vi "7HP v2.0 external control - EnFlo_Specific.vi"(6 "Datalog file path (full)":path, 7 "COM port":refnum<visa-resource-name>, 8 "Log data stream":bool, 9 "Set data rate (Hz)":u8(ring)=14 items=["1", "2", "4", "5", "8", "10", "16", "20", "25", "32", "40", "50", "64", "80", "100", "125", "160", "200", "250", "320", "400", "500", "625", "800", "1000"], 10 "N samples":u32=1000, 11 "Command":T2="D") -> (0 "Error":errorcluster, 1 "Returned data rate (Hz)":u16, 2 "Serial number":sgl, 3 "Data out":T3[](array[typedef]) {"Time stamp" format="%<%.6X\n%x>T"}, 4 "Rendezvous out":bool)   [LabVIEW 2021]
doc: "7HP test and configuration software.\nVersion 2.0\nSurrey Sensors Ltd.\n11/2023"
uses:
  ctls/7HP_Cmd (USB).ctl
  ctls/7HP_Data cluster.ctl
  Globals/Meas_global.vi
panel:
  in  "COM port 2":refnum<visa-resource-name>
  in  "Main":T1(tab)
  out "Subsystems ok":bool[](array[boolean])
  out "Pressure sensor values in range":bool[](array[boolean])
  out "Pressure sensor temperatures in range":bool[](array[boolean])
  out "Pressure sensor EEPROM checksums ok":bool[](array[boolean])
  out "P_raw_Azero":sgl[](array[numeric])
  out "n":u16
  out "Auto zero progBar":u16(slide) caption="Collecting samples, please maintain dP = 0" scale=0.0..1000.0
  out "Neural network binary (read-only)":string
  out "ANN checksum ok":bool
  out "Neural network checksum":u16 format="%04x"
  in  "EEPROM array 2":u16[](array[numeric])
  in  "EEPROM array":sgl[](array[numeric]) format="%#.3f"
  out "EEPROM checksum ok":bool
  out "EEPROM checksum":u16 format="%04x"
  out "received":bool
  out "sent":bool
  out "Neural network outputs":sgl[](array[numeric]) format="%#.2f"
  out "Frame errors":u32
  out "Checksum errors":u32
  in  "Stop Data":bool
  out "Rel. humidity (%)":sgl format="%#.2f"
  out "T_board (°C)":sgl format="%#.2f"
  out "T_external (°C)":sgl format="%#.2f"
  out "P_atmos (mbar)":sgl format="%#.2f"
  out "Checksum ok":bool
  out "Gyration vector (° / s)":sgl[](array[numeric]) format="%#.3f"
  out "Acceleration vector (g)":sgl[](array[numeric]) format="%#.3f"
  out "Pressures":sgl[][](graph)
  out "Stream enabled":bool
  out "Pitch (°)":sgl format="%.2f"
  out "Roll (°)":sgl format="%.2f"
  # "Paul Nathan 11/2023"
  # "Pressure sensor 0 EEPROM checksum okay"
  # "Pressure sensor 0 value in range"
  # "Pressure sensor 1 EEPROM checksum okay"
  # "Pressure sensor 1 value in range"
  # "Pressure sensor 2 EEPROM checksum okay"
  # "Pressure sensor 2 value in range"
  # "Pressure sensor 3 EEPROM checksum okay"
  # "Pressure sensor 3 value in range"
  # "Pressure sensor 4 EEPROM checksum okay"
  # "Pressure sensor 4 value in range"
  # "Pressure sensor 5 EEPROM checksum okay"
  # "Pressure sensor 5 value in range"
  # "Pressure sensor 6 EEPROM checksum okay"
  # "Pressure sensor 6 value in range"
  # "Environmental sensor present"
  # "Pressure sensor 0 temperature in range"
  # "Inertial sensor present"
  # "Pressure sensor 1 temperature in range"
  # "Accelerometer self test pass"
  # "Pressure sensor 2 temperature in range"
  # "Gyroscope self test pass"
  # "Pressure sensor 3 temperature in range"
  # "External thermistor value in range"
  # "Pressure sensor 4 temperature in range"
  # "MCU EEPROM checksum ok"
  # "Pressure sensor 5 temperature in range"
  # "Neural network enabled"
  # "Pressure sensor 6 temperature in range"
  # "Neural network integrity pass"
  # "%"
  # "P0 raw auto-zero"
  # "P1 raw auto-zero"
  # "P2 raw auto-zero"
  # "P3 raw auto-zero"
  # "P4 raw auto-zero"
  # "P5 raw auto-zero"
  # "P6 raw auto-zero"
  # "Power-up defaults"
  # "P0 raw auto-zero"
  # "Data rate (Hz)"
  # "P1 raw auto-zero"
  # "TTL streaming"
  # "P2 raw auto-zero"
  # "USB streaming"
  # "P3 raw auto-zero"
  # "TTL stream contains full data"
  # "P4 raw auto-zero"
  # "Accelerometer range mode"
  # "P5 raw auto-zero"
  # "Gyroscope range mode"
  # "P6 raw auto-zero"
  # "IMU rate mode"
  # "Atmospheric pressure offset (Pa)"
  # "HW trigger edge polarity"
  # "External thermistor temperature offset (°C)"
  # "Neural network enabled"
  # "Serial number"
  # "UVW coordinate system"
  # "TTL baud rate (bps)"
  # "Accelerometer vector magnitude scale factor"
  # "Gyroscope x component offset (deg / s)"
  # "Gyroscope y component offset (deg / s)"
  # "Gyroscope z component offset (deg / s)"
  # "||U|| (m/s)"
  # "Pitch (deg)"
  # "Yaw (deg)"
  # "U (m/s)"
  # "V (m/s)"
  # "W (m/s)"
  # "w_x"
  # "w_y"
  # "w_z"
  # "a_x"
  # "a_y"
  # "a_z"
  # "||U|| (m/s)"
  # "Pitch (deg)"
  # "Yaw (deg)"
  # "U (m/s)"
  # "V (m/s)"
  # "W (m/s)"
  # "w_x"
  # "w_y"
  # "w_z"
  # "a_x"
  # "a_y"
  # "a_z"
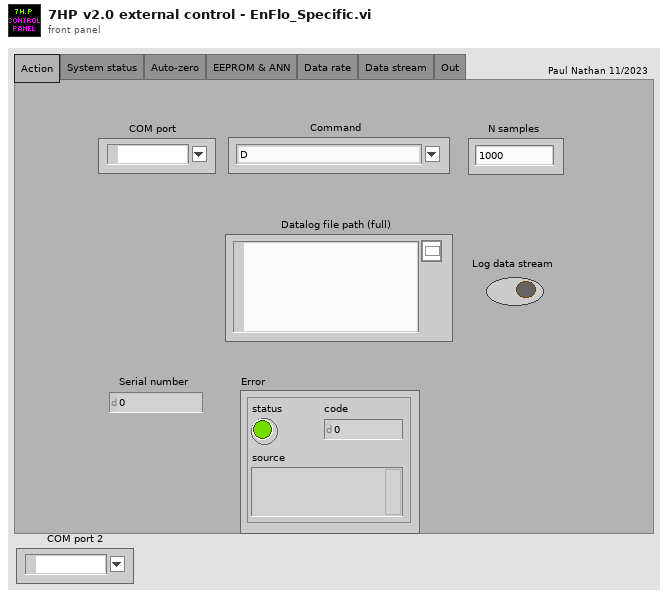
[diagram p1: front panel]
types:
  T1 = enum32{"Action", "System status", "Auto-zero", "EEPROM & ANN", "Data rate", "Data stream", "Out"}
  T2 = typedef "7HP_Cmd (USB).ctl" = string
  T3 = typedef "7HP_Data cluster.ctl" = cluster{"Time stamp":timestamp, "Pressures (Pa)":sgl[], "T_external (°C)":sgl, "P_atmos (mbar)":sgl, "T_board (°C)":sgl, "Rel. humidity (%)":sgl, "Acceleration vector (g)":sgl[], "Gyration vector (deg / s)":sgl[], "Neural network outputs":sgl[]}
  T4 = enum16{"open", "replace", "create", "open or create", "replace or create", "replace or create with confirmation"}
  T5 = typedef "Rendezvous RefNum" = refnum<k1>
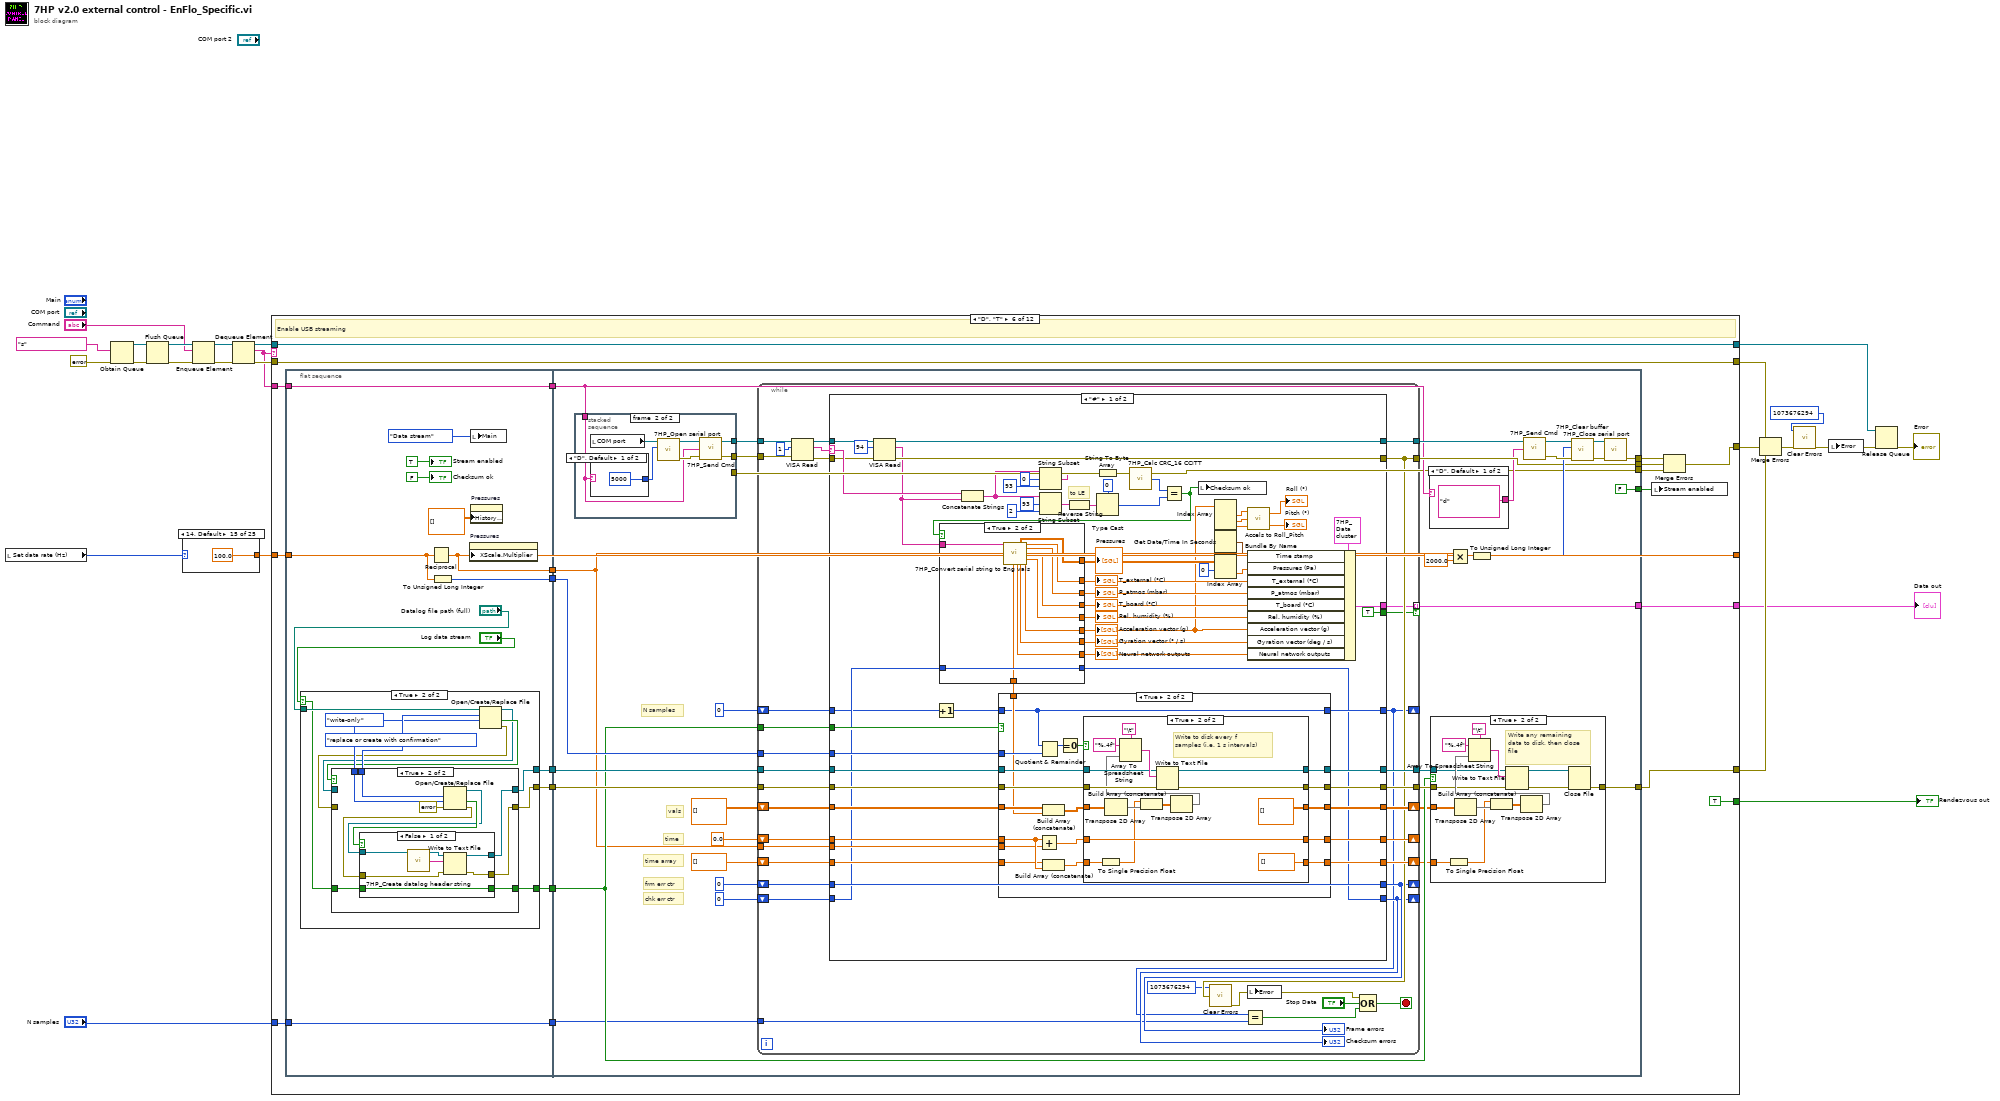
[diagram p0: block diagram]
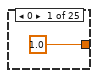
[diagram p2: hidden frame]
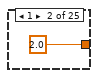
[diagram p3: hidden frame]
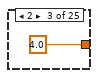
[diagram p4: hidden frame]
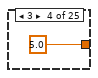
[diagram p5: hidden frame]
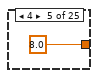
[diagram p6: hidden frame]
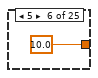
[diagram p7: hidden frame]
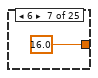
[diagram p8: hidden frame]
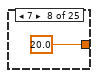
[diagram p9: hidden frame]
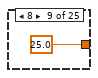
[diagram p10: hidden frame]
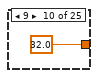
[diagram p11: hidden frame]
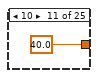
[diagram p12: hidden frame]
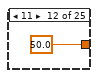
[diagram p13: hidden frame]
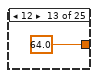
[diagram p14: hidden frame]
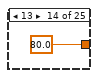
[diagram p15: hidden frame]
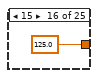
[diagram p16: hidden frame]
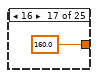
[diagram p17: hidden frame]
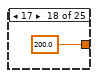
[diagram p18: hidden frame]
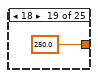
[diagram p19: hidden frame]
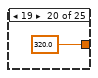
[diagram p20: hidden frame]
diagram:
  n1 = local read "Set data rate (Hz)"() -> (w4:u8)
  n2 = Obtain Queue(element data type=T2 "s" ("Combo Box"), error in (no error)=errorcluster {"status"=FALSE, "code"=0, "source"=""}) -> (queue out=w23:refnum<queue>, error out=w24:errorcluster)  [unwired: 3 in, 1 out]
  n3 = Flush Queue(queue=w23, error in (no error)=w24) -> (queue out=w19:refnum<queue>, error out=w20:errorcluster)  [unwired: 1 out]
  n4 = case shown="14, Default" w4 {
    tunnel: [1.0 2.0 4.0 5.0 8.0 10.0 16.0 20.0 25.0 32.0 40.0 50.0 64.0 80.0 100.0 125.0 160.0 200.0 250.0 320.0 400.0 500.0 625.0 800.0 1000.0] -> w5
    frame 0 {
    }
    frame 1 {
    }
    frame 2 {
    }
    frame 3 {
    }
    frame 4 {
    }
    frame 5 {
    }
    frame 6 {
    }
    frame 7 {
    }
    frame 8 {
    }
    frame 9 {
    }
    frame 10 {
    }
    frame 11 {
    }
    frame 12 {
    }
    frame 13 {
    }
    frame 14, Default {
    }
    frame 15 {
    }
    frame 16 {
    }
    frame 17 {
    }
    frame 18 {
    }
    frame 19 {
    }
    frame 20 {
    }
    frame 21 {
    }
    frame 22 {
    }
    frame 23 {
    }
    frame 24 {
    }
  }
  n5 = Enqueue Element(queue=w19, element="Command", error in (no error)=w20) -> (queue out=w18:refnum<queue>, error out=w17:errorcluster)  [unwired: 1 in, 1 out]
  n6 = Dequeue Element(queue=w18, error in (no error)=w17) -> (queue out=w15:refnum<queue>, element=w13:T2, error out=w14:errorcluster)  [unwired: 1 in, 1 out]
  n7 = case shown="\"D\", \"T\"" w13 {
    tunnel: [_ _ _ _ _ TRUE _ _ _ _ _ _] -> w1
    tunnel: w15 -> [w56 w95 w128 w193 w235 w303 w593 w617 w673 w709 w731 w735]
    tunnel: [w56 w95 w128 w193 w235 w303 w593 w617 w673 w709 w731 w735] -> w7
    tunnel: w14 -> [w55 w94 w127 w192 w234 w302 w592 w618 w674 w708 w730 w734]
    tunnel: [w55 w94 w127 w192 w234 w302 w592 w618 w674 w708 w730 w734] -> w12
    tunnel: w13 -> [w54 w93 w132 w190 w241 w301 w595 w623 w679 w707 _ _]
    tunnel: [w52 w91 w130 w188 w233 w289 w594 w616 w672 w705 errorcluster {"status"=FALSE, "code"=0, "source"=""} ("Error out") errorcluster {"status"=FALSE, "code"=0, "source"=""} ("Error out")] -> w11
    tunnel: [_ _ _ _ _ w299 _ _ _ _ _ _] -> w10
    tunnel: w5 -> [w51 w90 w129 w191 w238 w292 w590 _ _ w704 w728 w732]
    tunnel: [w51 w90 w129 w191 w238 w292 w590 w619 w675 w704 w728 w732] -> _
    tunnel: "N samples" -> [_ _ _ _ _ w287 _ _ _ _ _ _]
    tunnel: [_ _ _ _ _ w286 _ _ _ _ _ _] -> w2
    frame "S", "s" {
      # "Perform self-test and retrieve status bytes, Retrieve status bytes"
      n8 = flat-sequence {
        tunnel: w54 -> [w59]
        tunnel: [w59] -> w53
        tunnel: w53 -> [w65]
        tunnel: [w60] -> w52
        frame #0 {
          w58 = bool[] [] ("Pressure sensor EEPROM checksums ok")
          n9 = local write "Main"(T1."System status" ("Main")) -> ()
          "Pressure sensor EEPROM checksums ok" <- w58
          "Pressure sensor temperatures in range" <- w58
          "Pressure sensor values in range" <- w58
          "Subsystems ok" <- w58
        }
        frame #1 {
          w69 = 1 ("length (rest)")
          w77 = u8 0 ("byte count")
          n10 = local read "COM port"() -> (w66:refnum<visa-resource-name>)
          n11 = call "7HP_Open serial port.vi"("timeout (ms)"=u32 5000, "VISA resource name"=w66) -> ("Error out"=w87:errorcluster, "VISA resource name out"=w88:refnum<visa-resource-name>)  [unwired: 8 in]
          n12 = call "7HP_Send Cmd.vi"("Error In"=w87, "Operation"=w65, "Port"=w88) -> ("Error Out"=w85:errorcluster, "Port out"=w86:refnum<visa-resource-name>)  [unwired: 1 in]
          n13 = VISA Read(VISA resource name=w86, byte count=u32 4, error in (no error)=w85) -> (VISA resource name out=w83:refnum<visa-resource-name>, read buffer=w72:string, error out=w82:errorcluster)  [unwired: 1 out]
          n14 = call "7HP_Close serial port.vi"("Error in"=w82, "VISA resource name"=w83) -> ("Error out"=w60:errorcluster)  [unwired: 9 in]
          n15 = String Subset(string=w72, offset (0)=0, length (rest)=w69) -> (substring=w81:string)
          n16 = String Subset(string=w72, offset (0)=1, length (rest)=w69) -> (substring=w80:string)
          n17 = String Subset(string=w72, offset (0)=2 ("length (rest)"), length (rest)=w69) -> (substring=w79:string)
          n18 = String Subset(string=w72, offset (0)=3, length (rest)=w69) -> (substring=w78:string)
          n19 = Type Cast(type=w77, x=w81) -> (*(type *) &x=w76:u8)
          n20 = Type Cast(type=w77, x=w80) -> (*(type *) &x=w75:u8)
          n21 = Type Cast(type=w77, x=w79) -> (*(type *) &x=w74:u8)
          n22 = Type Cast(type=w77, x=w78) -> (*(type *) &x=w73:u8)
          n23 = Number To Boolean Array(number=w76) -> (Boolean array=w64:bool[])
          n24 = Number To Boolean Array(number=w75) -> (Boolean array=w63:bool[])
          n25 = Number To Boolean Array(number=w74) -> (Boolean array=w62:bool[])
          n26 = Number To Boolean Array(number=w73) -> (Boolean array=w61:bool[])
          n27 = local write "Pressure sensor EEPROM checksums ok"(w64) -> ()
          n28 = local write "Pressure sensor temperatures in range"(w63) -> ()
          n29 = local write "Pressure sensor values in range"(w62) -> ()
          n30 = local write "Subsystems ok"(w61) -> ()
        }
      }
    }
    frame "Z", "z" {
      # "Perform permanent auto-zero (write values to EEPROM), Perform temporary auto-zero"
      n31 = flat-sequence {
        tunnel: w93 -> [w99]
        tunnel: [w99] -> w92
        tunnel: w92 -> [w106]
        tunnel: [w102] -> w91
        frame #0 {
          n32 = local write "Main"(T1."Auto-zero" ("Main")) -> ()
          "P_raw_Azero" <- sgl[] [] ("P_raw_Azero")
          "Auto zero progBar" <- u16 0 ("Collecting samples, please maintain dP = 0")
        }
        frame #1 {
          n33 = local read "COM port"() -> (w107:refnum<visa-resource-name>)
          n34 = call "7HP_Open serial port.vi"("timeout (ms)"=u32 16000, "VISA resource name"=w107) -> ("Error out"=w113:errorcluster, "VISA resource name out"=w114:refnum<visa-resource-name>)  [unwired: 8 in]
          n35 = call "7HP_Send Cmd.vi"("Error In"=w113, "Operation"=w106, "Port"=w114) -> ("Error Out"=w111:errorcluster, "Port out"=w112:refnum<visa-resource-name>)  [unwired: 1 in]
          n36 = VISA Read(VISA resource name=w112, byte count=u32 28, error in (no error)=w111) -> (VISA resource name out=w109:refnum<visa-resource-name>, read buffer=w103:string, error out=w108:errorcluster)  [unwired: 1 out]
          n37 = for {
            N: 100 -> [_]
            shift-right: [w116] -> _
            shift-left: u16 0 -> [w117]
            n38 = Increment(x=w117) -> (x+1=w116:u16)
            "n" <- w116
            n39 = Wait (ms)(milliseconds to wait=u32 100) -> ()  [unwired: 1 out]
            n40 = local write "Auto zero progBar"(w116) -> ()
          }
          n41 = for {
            N: 7 -> [_]
            tunnel: [w120] -> w105 mode=indexing
            tunnel: w103 -> [w119]
            i -> [w126]
            w124 = 4 ("x")
            # "to BE"
            n42 = Multiply(x=w124, y=w126) -> (x*y=w125:i32)
            n43 = String Subset(string=w119, offset (0)=w125, length (rest)=w124) -> (substring=w123:string)
            n44 = Reverse String(1:w123) -> (0:w122:string)
            n45 = Type Cast(type=sgl 0.0 ("byte count"), x=w122) -> (*(type *) &x=w120:sgl)
          }
          n46 = call "7HP_Close serial port.vi"("Error in"=w108, "VISA resource name"=w109) -> ("Error out"=w102:errorcluster)  [unwired: 9 in]
          n47 = local write "P_raw_Azero"(w105) -> ()
        }
      }
    }
    frame "R" {
      # "Read all EEPROM values"
      n48 = flat-sequence {
        tunnel: w132 -> [w138]
        tunnel: [w138] -> w131
        tunnel: w131 -> [w170]
        tunnel: [w168] -> w130
        frame #0 {
          n49 = local write "EEPROM checksum ok"(FALSE ("Chk ok")) -> ()
          n50 = local write "EEPROM checksum"(u16 0 ("EEPROM checksum")) -> ()
          n51 = local write "EEPROM array"(sgl[] [] ("EEPROM array")) -> ()
          n52 = local write "EEPROM array 2"(u16[] [] ("EEPROM array 2")) -> ()
          n53 = local write "Main"(T1."EEPROM & ANN" ("Main")) -> ()
        }
        frame #1 {
          # "to BE"
          # "to BE"
          n54 = local read "COM port"() -> (w171:refnum<visa-resource-name>)
          n55 = call "7HP_Open serial port.vi"("timeout (ms)"=u32 5000, "VISA resource name"=w171) -> ("Error out"=w177:errorcluster, "VISA resource name out"=w178:refnum<visa-resource-name>)  [unwired: 8 in]
          n56 = call "7HP_Send Cmd.vi"("Error In"=w177, "Operation"=w170, "Port"=w178) -> ("Error Out"=w175:errorcluster, "Port out"=w176:refnum<visa-resource-name>)  [unwired: 1 in]
          n57 = VISA Read(VISA resource name=w176, byte count=u32 73, error in (no error)=w175) -> (VISA resource name out=w173:refnum<visa-resource-name>, read buffer=w144:string, error out=w172:errorcluster)  [unwired: 1 out]
          n58 = call "7HP_Close serial port.vi"("Error in"=w172, "VISA resource name"=w173) -> ("Error out"=w168:errorcluster)  [unwired: 9 in]
          n59 = String Subset(string=w144, offset (0)=0, length (rest)=60 ("length (rest)")) -> (substring=w167:string)
          n60 = String Subset(string=w144, offset (0)=60, length (rest)=2 ("length (rest)")) -> (substring=w158:string)
          n61 = String Subset(string=w144, offset (0)=62, length (rest)=9 ("length (rest)")) -> (substring=w153:string)
          n62 = String Subset(string=w144, offset (0)=71, length (rest)=2 ("length (rest)")) -> (substring=w145:string)
          n63 = String Subset(string=w144, offset (0)=0, length (rest)=71 ("length (rest)")) -> (substring=w141:string)
          n64 = for {
            N: 15 -> [_]
            tunnel: [w183] -> w139 mode=indexing
            tunnel: w167 -> [w182]
            i -> [w187]
            w185 = 4 ("x")
            # "to BE"
            n65 = Multiply(x=w185, y=w187) -> (x*y=w186:i32)
            n66 = String Subset(string=w182, offset (0)=w186, length (rest)=w185) -> (substring=w181:string)
            n67 = Reverse String(1:w181) -> (0:w180:string)
            n68 = Type Cast(type=sgl 0.0 ("byte count"), x=w180) -> (*(type *) &x=w183:sgl)
          }
          n69 = Reverse String(1:w158) -> (0:w164:string)
          n70 = Reverse String(1:w145) -> (0:w149:string)
          n71 = String To Byte Array(string=w141) -> (unsigned byte array=w152:u8[])
          n72 = call "7HP_Calc CRC_16 CCITT.vi"("Data bytes"=w152) -> ("CRC_16-CCITT"=w151:u16)  [unwired: 1 in]
          n73 = Type Cast(type=u16 0 ("byte count"), x=w164) -> (*(type *) &x=w157:u16)
          n74 = Type Cast(type=u16 0 ("byte count"), x=w149) -> (*(type *) &x=w140:u16)
          n75 = String To Byte Array(string=w153) -> (unsigned byte array=w156:u8[])
          n76 = To Unsigned Word Integer(number=w156) -> (unsigned 16bit integer=w154:u16[])
          n77 = Equal?(x=w140, y=w151) -> (x = y?=w150:bool)
          n78 = Build Array (concatenate)(w157, w154) -> (w155:u16[])
          n79 = local write "EEPROM checksum ok"(w150) -> ()
          n80 = local write "EEPROM array"(w139) -> ()
          n81 = local write "EEPROM array 2"(w155) -> ()
          n82 = local write "EEPROM checksum"(w140) -> ()
        }
      }
    }
    frame "u" {
      # "Read ANN bytes"
      n83 = flat-sequence {
        tunnel: w190 -> [w194]
        tunnel: [w194] -> w189
        tunnel: w189 -> [w225]
        tunnel: [w201] -> w188
        frame #0 {
          n84 = local write "Neural network binary (read-only)"("") -> ()
          n85 = local write "ANN checksum ok"(FALSE ("ANN checksum ok")) -> ()
          n86 = local write "Neural network checksum"(u16 0 ("Neural network checksum")) -> ()
          n87 = local write "Main"(T1."EEPROM & ANN" ("Main")) -> ()
        }
        frame #1 {
          # "to BE"
          # "to BE"
          n88 = local read "COM port"() -> (w228:refnum<visa-resource-name>)
          n89 = call "7HP_Open serial port.vi"("timeout (ms)"=u32 5000, "VISA resource name"=w228) -> ("Error out"=w231:errorcluster, "VISA resource name out"=w232:refnum<visa-resource-name>)  [unwired: 8 in]
          n90 = call "7HP_Send Cmd.vi"("Error In"=w231, "Operation"=w225, "Port"=w232) -> ("Error Out"=w229:errorcluster, "Port out"=w230:refnum<visa-resource-name>)  [unwired: 1 in]
          n91 = VISA Read(VISA resource name=w230, byte count=u32 2, error in (no error)=w229) -> (VISA resource name out=w224:refnum<visa-resource-name>, read buffer=w207:string, error out=w223:errorcluster)  [unwired: 1 out]
          n92 = Reverse String(1:w207) -> (0:w218:string)
          n93 = Type Cast(type=u16 0 ("byte count"), x=w218) -> (*(type *) &x=w219:u16)
          n94 = Subtract(x=w219, y=u16 2) -> (x-y=w200:u16)
          n95 = VISA Read(VISA resource name=w224, byte count=w200, error in (no error)=w223) -> (VISA resource name out=w221:refnum<visa-resource-name>, read buffer=w217:string, error out=w222:errorcluster)  [unwired: 1 out]
          n96 = Concatenate Strings(w207, w217) -> (w204:string)
          "Neural network binary (read-only)" <- w204
          n97 = String Length(string=w204) -> (length=w206:i32)
          n98 = Subtract(x=w206, y=2) -> (x-y=w203:i32)
          n99 = call "7HP_Close serial port.vi"("Error in"=w222, "VISA resource name"=w221) -> ("Error out"=w201:errorcluster)  [unwired: 9 in]
          n100 = String Subset(string=w204, offset (0)=w203, length (rest)=2 ("length (rest)")) -> (substring=w213:string)
          n101 = String Subset(string=w204, offset (0)=0, length (rest)=w203) -> (substring=w212:string)
          n102 = Reverse String(1:w213) -> (0:w214:string)
          n103 = String To Byte Array(string=w212) -> (unsigned byte array=w216:u8[])
          n104 = call "7HP_Calc CRC_16 CCITT.vi"("Data bytes"=w216) -> ("CRC_16-CCITT"=w215:u16)  [unwired: 1 in]
          n105 = Type Cast(type=u16 0 ("byte count"), x=w214) -> (*(type *) &x=w202:u16)
          "Neural network checksum" <- w202
          n106 = Equal?(x=w202, y=w215) -> (x = y?=→"ANN checksum ok":bool)
        }
      }
    }
    frame "W" {
      # "Write all EEPROM values (including new checksum)"
      n107 = flat-sequence {
        tunnel: w241 -> [w251]
        tunnel: [w251] -> w240
        tunnel: ["EEPROM array"] -> w239
        tunnel: [w245] -> w237
        tunnel: [w246] -> w236
        tunnel: w240 -> [w273]
        tunnel: w239 -> [w268]
        tunnel: [w267] -> w233
        tunnel: w237 -> [w259]
        tunnel: w236 -> [w257]
        frame #0 {
          n108 = local write "Main"(T1."EEPROM & ANN" ("Main")) -> ()
          n109 = Split 1D Array(array="EEPROM array 2", index=1) -> (first subarray=w248:u16[], second subarray=w247:u16[])
          n110 = Index Array(array=w248, index=0) -> (element=w245:u16)
          n111 = To Unsigned Byte Integer(number=w247) -> (unsigned 8bit integer=w246:u8[])
        }
        frame #1 {
          # "to LE"
          # "to LE"
          n112 = local read "COM port"() -> (w274:refnum<visa-resource-name>)
          n113 = for {
            N: 15 -> [_]
            tunnel: w268 -> [w280] mode=indexing
            shift-right: [w281] -> w263
            shift-left: "" -> [w282]
            # "to LE"
            n114 = Type Cast(type="", x=w280) -> (*(type *) &x=w279:string)
            n115 = Reverse String(1:w279) -> (0:w278:string)
            n116 = Concatenate Strings(w282, w278) -> (w281:string)
          }
          n117 = Type Cast(type="", x=w259) -> (*(type *) &x=w261:string)
          n118 = Reverse String(1:w261) -> (0:w258:string)
          n119 = Byte Array To String(unsigned byte array=w257) -> (string=w256:string)
          n120 = call "7HP_Open serial port.vi"("timeout (ms)"=u32 5000, "VISA resource name"=w274) -> ("Error out"=w275:errorcluster, "VISA resource name out"=w276:refnum<visa-resource-name>)  [unwired: 8 in]
          n121 = Concatenate Strings(w263, w258, w256) -> (w262:string)
          n122 = String To Byte Array(string=w262) -> (unsigned byte array=w255:u8[])
          n123 = call "7HP_Calc CRC_16 CCITT.vi"("Data bytes"=w255) -> ("CRC_16-CCITT"=w254:u16)  [unwired: 1 in]
          "EEPROM checksum" <- w254
          n124 = Type Cast(type="", x=w254) -> (*(type *) &x=w253:string)
          n125 = Reverse String(1:w253) -> (0:w252:string)
          n126 = Concatenate Strings(w262, w252) -> (w266:string)
          n127 = call "7HP_Send Cmd + Data.vi"("Error In"=w275, "Data"=w266, "Operation"=w273, "Port"=w276) -> ("Error Out"=w264:errorcluster, "Port out"=w265:refnum<visa-resource-name>)  [unwired: 1 in]
          n128 = call "7HP_Close serial port.vi"("Error in"=w264, "VISA resource name"=w265) -> ("Error out"=w267:errorcluster)  [unwired: 9 in]
          "EEPROM checksum ok" <- TRUE ("Chk ok")
        }
      }
    }
    frame "D", "T" {
      # "Enable USB streaming"
      n129 = flat-sequence {
        tunnel: w301 -> [w317]
        tunnel: [w317] -> w300
        tunnel: [w314] -> w298
        tunnel: [w313] -> w297
        tunnel: [w312] -> w296
        tunnel: w292 -> [w307]
        tunnel: [w306] -> w295
        tunnel: [w308] -> w294
        tunnel: [w304] -> w288
        tunnel: w287 -> [w304]
        tunnel: w300 -> [w359]
        tunnel: [w389] -> w290
        tunnel: [w388] -> w299
        tunnel: w298 -> [w385]
        tunnel: w297 -> [w384]
        tunnel: w296 -> [w386]
        tunnel: w295 -> [w368]
        tunnel: w294 -> [w378]
        tunnel: [FALSE] -> w293
        tunnel: [w363] -> w291
        tunnel: w288 -> [w360]
        tunnel: [w357] -> w286
        tunnel: [w356] -> w285
        frame #0 {
          n130 = case shown="True" "Log data stream" {
            selector: "Log data stream" -> [w318 w321]
            tunnel: "Datalog file path (full)" -> [_ w330]
            tunnel: [refnum<file> refnum ("refnum out") w327] -> w314
            tunnel: [errorcluster {"status"=FALSE, "code"=0, "source"=""} ("error out") w326] -> w313
            tunnel: [w318 w322] -> w308
            frame False {
            }
            frame True {
              w328 = enum16{"read/write", "read-only", "write-only"}."write-only" ("access (0:read/write)")
              w329 = T4."replace or create with confirmation" ("operation (0:open)")
              n131 = Open/Create/Replace File(file path (use dialog)=w330, operation (0:open)=w329, access (0:read/write)=w328) -> (refnum out=w323:refnum<file>, cancelled=w325:bool, error out=w324:errorcluster)  [unwired: 3 in]
              n132 = case shown="True" w325 {
                tunnel: w329 -> [_ w346]
                tunnel: w328 -> [_ w345]
                tunnel: w324 -> [w334 _]
                tunnel: [w332 w340] -> w327
                tunnel: [w333 w341] -> w326
                tunnel: w323 -> [w335 _]
                tunnel: [w331 w338] -> w322
                tunnel: w321 -> [w331 w337]
                frame False {
                  n133 = call "7HP_Create datalog header string.vi"() -> ("Datalog header string"=w336:string)  [unwired: 1 in]
                  n134 = Write to Text File(file (use dialog)=w335, text=w336, error in=w334) -> (refnum out=w332:refnum<file>, error out=w333:errorcluster)  [unwired: 1 in, 1 out]
                }
                frame True {
                  n135 = Open/Create/Replace File(error in=errorcluster {"status"=FALSE, "code"=0, "source"=""}, operation (0:open)=w346, access (0:read/write)=w345) -> (refnum out=w343:refnum<file>, cancelled=w344:bool, error out=w342:errorcluster)  [unwired: 3 in]
                  n136 = case shown="False" w344 {
                    tunnel: w343 -> [w351 _]
                    tunnel: w342 -> [w350 _]
                    tunnel: [w349 errorcluster {"status"=FALSE, "code"=0, "source"=""} ("error out")] -> w341
                    tunnel: [w348 refnum<file> refnum ("t")] -> w340
                    tunnel: [w347 w353] -> w338
                    tunnel: w337 -> [w347 _]
                    frame False {
                      n137 = call "7HP_Create datalog header string.vi"() -> ("Datalog header string"=w352:string)  [unwired: 1 in]
                      n138 = Write to Text File(file (use dialog)=w351, text=w352, error in=w350) -> (refnum out=w348:refnum<file>, error out=w349:errorcluster)  [unwired: 1 in, 1 out]
                    }
                    frame True {
                      w353 = FALSE ("Log data stream")
                      n139 = local write "Log data stream"(w353) -> ()
                    }
                  }
                }
              }
            }
          }
          n140 = Reciprocal(x=w307) -> (1/x=w306:dbl)
          n141 = To Unsigned Long Integer(number=w307) -> (unsigned 32bit integer=w312:u32)
          n142 = property on="Pressures" class="WFChart (strict)"("XScale.Multiplier"=w306) -> ()  [unwired: 2 in, 2 out]
          n143 = local write "Main"(T1."Data stream" ("Main")) -> ()
          n144 = property on="Pressures" class="WFChart (strict)"("History Data"=sgl[][] []) -> ()  [unwired: 2 in, 2 out]
          "Checksum ok" <- FALSE ("Checksum ok")
          "Stream enabled" <- TRUE ("Stream enabled")
        }
        frame #1 {
          # "N samples"
          # "chk err ctr"
          # "frm err ctr"
          # "vals"
          # "time"
          # "time array"
          n145 = stacked-sequence {
            tunnel: [_ w397] -> w377
            tunnel: [_ w395] -> w376
            tunnel: w359 -> [_ w393]
            tunnel: [w390 _] -> w356
            frame #0 {
              # "Wait here until all acq. devs. are ready."
              n146 = global read "Meas_global.vi" "Acquisition Rendezvous"() -> (w392:T5)
              n147 = call <vilib>:"Wait at Rendezvous.vi"("ms timeout (-1)"=60000, "rendezvous"=w392) -> ("error out"=w390:errorcluster)  [unwired: 3 in, 2 out]
            }
            frame #1 {
              n148 = local read "COM port"() -> (w399:refnum<visa-resource-name>)
              n149 = case shown="\"D\", Default" w393 {
                tunnel: [u32 5000 ("timeout (ms)") u32 15000 ("timeout (ms)")] -> w394
                frame "D", Default {
                }
                frame "T" {
                }
              }
              n150 = call "7HP_Open serial port.vi"("timeout (ms)"=w394, "VISA resource name"=w399) -> ("Error out"=w396:errorcluster, "VISA resource name out"=w398:refnum<visa-resource-name>)  [unwired: 8 in]
              n151 = call "7HP_Send Cmd.vi"("Error In"=w396, "Operation"=w393, "Port"=w398) -> ("Error Out"=w395:errorcluster, "Port out"=w397:refnum<visa-resource-name>)  [unwired: 1 in]
            }
          }
          n152 = while {
            tunnel: [w415] -> w363
            tunnel: w377 -> [w417]
            tunnel: [w434] -> w375
            shift-right: [w408] -> _
            shift-left: u32 0 -> [w431]
            tunnel: w386 -> [w430]
            tunnel: w385 -> [w429]
            tunnel: w384 -> [w428]
            tunnel: [w427] -> w383
            tunnel: [w426] -> w382
            shift-right: [w425] -> w365
            shift-left: sgl[][] [] -> [w424]
            shift-right: [w421] -> _
            shift-left: 0.0 ("Numeric") -> [w423]
            tunnel: w368 -> [w422]
            shift-right: [w419] -> w364
            shift-left: dbl[] [] -> [w420]
            tunnel: w378 -> [w418]
            tunnel: w376 -> [w416]
            shift-right: [w410] -> _
            shift-left: u32 0 -> [w412]
            shift-right: [w409] -> _
            shift-left: u32 0 -> [w411]
            tunnel: w360 -> [w407]
            tunnel: [w405] -> w357 mode=indexing if=w404
            stop <- w432 stop-if-true
            n153 = VISA Read(VISA resource name=w417, byte count=u32 1, error in (no error)=w416) -> (VISA resource name out=w436:refnum<visa-resource-name>, read buffer=w437:string, error out=w435:errorcluster)  [unwired: 1 out]
            n154 = case shown="\"#\"" w437 {
              selector: w437 -> [w480 _]
              tunnel: w436 -> [w466 w573]
              tunnel: [w496 w574] -> w415
              tunnel: w435 -> [w465 w574]
              tunnel: [w497 w573] -> w434
              tunnel: w431 -> [w459 w572]
              tunnel: [w495 w572] -> w408
              tunnel: w430 -> [w494 _]
              tunnel: w429 -> [w493 w571]
              tunnel: w428 -> [w492 w570]
              tunnel: [w491 w570] -> w427
              tunnel: [w490 w571] -> w426
              tunnel: [w489 w569] -> w425
              tunnel: w424 -> [w488 w569]
              tunnel: w423 -> [w487 w568]
              tunnel: w422 -> [w486 _]
              tunnel: [w485 w568] -> w421
              tunnel: w420 -> [w484 w567]
              tunnel: [w483 w567] -> w419
              tunnel: w418 -> [w482 _]
              tunnel: w412 -> [w481 w566]
              tunnel: w411 -> [w461 w565]
              tunnel: [w481 w564] -> w410
              tunnel: [w460 w565] -> w409
              tunnel: [w454 _] -> w405
              tunnel: [TRUE FALSE] -> w404
              frame "#" {
                # "to LE"
                n155 = VISA Read(VISA resource name=w466, byte count=u32 94, error in (no error)=w465) -> (VISA resource name out=w497:refnum<visa-resource-name>, read buffer=w464:string, error out=w496:errorcluster)  [unwired: 1 out]
                n156 = Increment(x=w459) -> (x+1=w458:u32)
                n157 = Concatenate Strings(w480, w464) -> (w468:string)
                n158 = String Subset(string=w468, offset (0)=0, length (rest)=93 ("length (rest)")) -> (substring=w467:string)
                n159 = String Subset(string=w468, offset (0)=93, length (rest)=2 ("length (rest)")) -> (substring=w474:string)
                n160 = Reverse String(1:w474) -> (0:w473:string)
                n161 = String To Byte Array(string=w467) -> (unsigned byte array=w478:u8[])
                n162 = Type Cast(type=u16 0 ("length (rest)"), x=w473) -> (*(type *) &x=w472:u16)
                n163 = call "7HP_Calc CRC_16 CCITT.vi"("Data bytes"=w478) -> ("CRC_16-CCITT"=w471:u16)  [unwired: 1 in]
                n164 = Equal?(x=w471, y=w472) -> (x = y?=w462:bool)
                n165 = case shown="True" w462 {
                  tunnel: w464 -> [_ w516]
                  tunnel: [w504 w515] -> w456
                  tunnel: [w500 w514] -> w450
                  tunnel: [w500 w513] -> w449
                  tunnel: [w500 w512] -> w448
                  tunnel: [w500 w511] -> w447
                  tunnel: [w499 w510] -> w439
                  tunnel: [w499 w509] -> w446
                  tunnel: [w501 w507] -> w463
                  tunnel: w461 -> [w503 w508]
                  tunnel: [w502 w508] -> w460
                  tunnel: [sgl[] [nan, nan, nan, nan, nan, nan] w506] -> w445
                  frame False {
                    w505 = sgl[] [nan, nan, nan, nan, nan, nan, nan]
                    w500 = sgl nan
                    w499 = sgl[] [nan, nan, nan]
                    n166 = Increment(x=w503) -> (x+1=w502:u32)
                    n167 = Build Array (concatenate)(w505, w500, w500, w500, w500, w499, w499) -> (w501:sgl[])
                    n168 = Build Array(w505) -> (w504:sgl[][])
                  }
                  frame True {
                    n169 = call "7HP_Convert serial string to Eng vals.vi"("Serial buffer string (excluding FrameChar)"=w516) -> ("All vals"=w507:sgl[], "ANN output vector"=w506:sgl[], "Pressures"=w515:sgl[][], "Gyration vector (deg / s)"=w509:sgl[], "External thermistor temperature (deg C)"=w514:sgl, "Atmospheric pressure (mbar)"=w513:sgl, "Env. sensor die temperature (deg C)"=w512:sgl, "Relative humidity (%)"=w511:sgl, "Acceleration vector (g)"=w510:sgl[])  [unwired: 10 in]
                  }
                }
                "Pressures" <- w456
                "Acceleration vector (g)" <- w439
                "Gyration vector (° / s)" <- w446
                "P_atmos (mbar)" <- w449
                "T_external (°C)" <- w450
                "T_board (°C)" <- w448
                "Rel. humidity (%)" <- w447
                "Neural network outputs" <- w445
                n170 = case shown="True" w482 {
                  tunnel: w458 -> [w522 w523]
                  tunnel: [w522 w523] -> w495
                  tunnel: w494 -> [_ w541]
                  tunnel: w463 -> [_ w527]
                  tunnel: w493 -> [w520 w538]
                  tunnel: w492 -> [w521 w537]
                  tunnel: [w521 w536] -> w491
                  tunnel: [w520 w535] -> w490
                  tunnel: w488 -> [w519 w528]
                  tunnel: [w519 w534] -> w489
                  tunnel: w487 -> [w518 w531]
                  tunnel: w486 -> [_ w530]
                  tunnel: [w518 w533] -> w485
                  tunnel: w484 -> [w517 w529]
                  tunnel: [w517 w532] -> w483
                  frame False {
                  }
                  frame True {
                    n171 = Add(x=w531, y=w530) -> (x+y=w526:dbl)
                    n172 = Quotient & Remainder(x=w523, y=w541) -> (x-y*floor(x/y)=w540:u32)  [unwired: 1 out]
                    n173 = Build Array (concatenate)(w528, w527) -> (w524:sgl[][])
                    n174 = Build Array (concatenate)(w529, w531) -> (w525:dbl[])
                    n175 = Equal To 0?(x=w540) -> (x = 0?=w539:bool)
                    n176 = case shown="True" w539 {
                      tunnel: w538 -> [w545 w559]
                      tunnel: w537 -> [w546 w558]
                      tunnel: [w546 w557] -> w536
                      tunnel: [w545 w556] -> w535
                      tunnel: w524 -> [w543 w551]
                      tunnel: [w543 sgl[][] []] -> w534
                      tunnel: w526 -> [w544 w554]
                      tunnel: [w544 w554] -> w533
                      tunnel: w525 -> [w542 w553]
                      tunnel: [w542 dbl[] []] -> w532
                      frame False {
                      }
                      frame True {
                        # "Write to disk every f samples (i.e. 1 s intervals)"
                        n177 = To Single Precision Float(number=w553) -> (single precision float=w547:sgl[])
                        n178 = Transpose 2D Array(2D array=w551) -> (transposed array=w550:sgl[][])
                        n179 = Build Array (concatenate)(w547, w550) -> (w549:sgl[][])
                        n180 = Transpose 2D Array(2D array=w549) -> (transposed array=w548:sgl[][])
                        n181 = Array To Spreadsheet String(delimiter (Tab)="\t", array=w548, 3:"%.4f" ("format string")) -> (spreadsheet string=w562:string)
                        n182 = Write to Text File(file (use dialog)=w559, text=w562, error in=w558) -> (refnum out=w556:refnum<file>, error out=w557:errorcluster)  [unwired: 1 in, 1 out]
                      }
                    }
                  }
                }
                n183 = local write "Checksum ok"(w462) -> ()
                n184 = Index Array(array=w439) -> (element #1=w444:sgl, element #2=w443:sgl, element #3=w442:sgl)  [unwired: 3 in]
                n185 = Get Date/Time In Seconds() -> (seconds since 1Jan1904=w452:timestamp)
                n186 = Index Array(array=w456, index (row)=0) -> (element=w451:sgl[])  [unwired: 1 in]
                n187 = call "Accels to Roll_Pitch.vi"("az"=w442, "ay"=w443, "ax"=w444) -> ("Pitch (deg)"=→"Pitch (°)":sgl, "Roll (deg)"=→"Roll (°)":sgl)
                n188 = Bundle By Name(cluster=T3 {"Time stamp"=timestamp(0 s since 1904-01-01), "Pressures (Pa)"=[], "T_external (°C)"=0.0, "P_atmos (mbar)"=0.0, "T_board (°C)"=0.0, "Rel. humidity (%)"=0.0, "Acceleration vector (g)"=[], "Gyration vector (deg / s)"=[], "Neural network outputs"=[]} ("Data cluster 7HP"), "Time stamp"=w452, "Pressures (Pa)"=w451, "T_external (°C)"=w450, "P_atmos (mbar)"=w449, "T_board (°C)"=w448, "Rel. humidity (%)"=w447, "Acceleration vector (g)"=w439, "Gyration vector (deg / s)"=w446, "Neural network outputs"=w445) -> (w454:T3)
              }
              frame Default {
                # "Frame error"
                n189 = Increment(x=w566) -> (x+1=w564:u32)
              }
            }
            "Checksum errors" <- w409
            "Frame errors" <- w410
            n190 = call <vilib>:"Clear Errors.vi"("error in (no error)"=w415, "specific error code to clear (0: all)"=1073676294) -> ("error out"=w414:errorcluster)  [unwired: 4 in, 1 out]
            n191 = Equal?(x=w408, y=w407) -> (x = y?=w406:bool)
            n192 = local write "Error"(w414) -> ()
            n193 = Compound Arithmetic op=OR(w414, "Stop Data", w406) -> (w432:bool)
          }
          n194 = case shown="\"D\", Default" w359 {
            tunnel: [T2 "d" ("Combo Box") T2 "t" ("Combo Box")] -> w358
            frame "D", Default {
            }
            frame "T" {
            }
          }
          n195 = case shown="True" w378 {
            tunnel: [w575 w589] -> w388
            tunnel: w383 -> [w575 w581]
            tunnel: w382 -> [_ w582]
            tunnel: w365 -> [_ w580]
            tunnel: w364 -> [_ w579]
            frame False {
            }
            frame True {
              # "Write any remaining data to disk, then close file"
              n196 = To Single Precision Float(number=w579) -> (single precision float=w576:sgl[])
              n197 = Transpose 2D Array(2D array=w580) -> (transposed array=w586:sgl[][])
              n198 = Build Array (concatenate)(w576, w586) -> (w587:sgl[][])
              n199 = Transpose 2D Array(2D array=w587) -> (transposed array=w588:sgl[][])
              n200 = Array To Spreadsheet String(delimiter (Tab)="\t", array=w588, 3:"%.4f" ("format string")) -> (spreadsheet string=w583:string)
              n201 = Write to Text File(file (use dialog)=w582, text=w583, error in=w581) -> (refnum out=w578:refnum<file>, error out=w577:errorcluster)  [unwired: 1 in, 1 out]
              n202 = Close File(refnum=w578, error in=w577) -> (error out=w589:errorcluster)  [unwired: 1 out]
            }
          }
          n203 = Multiply(x=w368, y=2000.0) -> (x*y=w369:dbl)
          n204 = To Unsigned Long Integer(number=w369) -> (unsigned 32bit integer=w366:u32)
          n205 = call "7HP_Send Cmd.vi"("Operation"=w358, "Port"=w375) -> ("Error Out"=w372:errorcluster, "Port out"=w373:refnum<visa-resource-name>)  [unwired: 2 in]
          n206 = call "7HP_Clear buffer.vi"("Error in"=w372, "dt for timeout (ms)"=w366, "VISA resource name in"=w373) -> ("Error out"=w370:errorcluster, "VISA resource name out"=w371:refnum<visa-resource-name>)  [unwired: 3 in]
          n207 = call "7HP_Close serial port.vi"("Error in"=w370, "VISA resource name"=w371) -> ("Error out"=w389:errorcluster)  [unwired: 9 in]
        }
      }
      n208 = local write "Stream enabled"(w293) -> ()
      n209 = Merge Errors(w290, w291, w285) -> (w289:errorcluster)
    }
    frame "d", "t" {
      # "Disable USB streaming"
      n210 = flat-sequence {
        tunnel: [w603] -> w596
        tunnel: w595 -> [w603]
        tunnel: w590 -> [w602]
        tunnel: [w597] -> w591
        tunnel: w596 -> [w611]
        tunnel: [w610] -> w594
        tunnel: w591 -> [w605]
        frame #0 {
          n211 = Reciprocal(x=w602) -> (1/x=w601:dbl)
          n212 = disable-structure shown="Disabled" {
            frame Disabled {
              n213 = local write "Main"(T1."Data stream" ("Main")) -> ()
            }
            frame Enabled {
            }
          }
          n214 = To Single Precision Float(number=w601) -> (single precision float=w598:sgl)
          n215 = Multiply(x=w598, y=sgl 2000.0) -> (x*y=w599:sgl)
          n216 = To Unsigned Long Integer(number=w599) -> (unsigned 32bit integer=w597:u32)
        }
        frame #1 {
          n217 = local read "COM port"() -> (w612:refnum<visa-resource-name>)
          n218 = call "7HP_Open serial port.vi"("timeout (ms)"=u32 5000, "VISA resource name"=w612) -> ("Error out"=w613:errorcluster, "VISA resource name out"=w614:refnum<visa-resource-name>)  [unwired: 8 in]
          n219 = call "7HP_Send Cmd.vi"("Error In"=w613, "Operation"=w611, "Port"=w614) -> ("Error Out"=w609:errorcluster, "Port out"=w607:refnum<visa-resource-name>)  [unwired: 1 in]
          n220 = call "7HP_Clear buffer.vi"("Error in"=w609, "dt for timeout (ms)"=w605, "VISA resource name in"=w607) -> ("Error out"=w608:errorcluster, "VISA resource name out"=w606:refnum<visa-resource-name>)  [unwired: 3 in]
          n221 = call "7HP_Close serial port.vi"("Error in"=w608, "VISA resource name"=w606) -> ("Error out"=w610:errorcluster)  [unwired: 9 in]
        }
      }
    }
    frame "F" {
      # "Set data rate"
      n222 = flat-sequence {
        tunnel: w623 -> [w627]
        tunnel: [w627] -> w622
        tunnel: w622 -> [w632]
        tunnel: [w631] -> w621
        tunnel: [w630] -> w620
        tunnel: [w670] -> w619
        tunnel: w621 -> [w670]
        tunnel: w620 -> [w668]
        tunnel: [w668] -> w616
        frame #0 {
          n223 = local write "Returned data rate (Hz)"(u16 0 ("Returned data rate (Hz)")) -> ()
          n224 = local write "received"(FALSE ("sent")) -> ()
          n225 = local write "Main"(T1."Data rate" ("Main")) -> ()
          n226 = local write "sent"(FALSE ("sent")) -> ()
        }
        frame #1 {
          # "to LE"
          n227 = case shown="14, Default" "Set data rate (Hz)" {
            tunnel: [1.0 2.0 4.0 5.0 8.0 10.0 16.0 20.0 25.0 32.0 40.0 50.0 64.0 80.0 100.0 125.0 160.0 200.0 250.0 320.0 400.0 500.0 625.0 800.0 1000.0] -> w631
            frame 0 {
            }
            frame 1 {
            }
            frame 2 {
            }
            frame 3 {
            }
            frame 4 {
            }
            frame 5 {
            }
            frame 6 {
            }
            frame 7 {
            }
            frame 8 {
            }
            frame 9 {
            }
            frame 10 {
            }
            frame 11 {
            }
            frame 12 {
            }
            frame 13 {
            }
            frame 14, Default {
            }
            frame 15 {
            }
            frame 16 {
            }
            frame 17 {
            }
            frame 18 {
            }
            frame 19 {
            }
            frame 20 {
            }
            frame 21 {
            }
            frame 22 {
            }
            frame 23 {
            }
            frame 24 {
            }
          }
          n228 = local read "COM port"() -> (w635:refnum<visa-resource-name>)
          n229 = To Unsigned Word Integer(number=w631) -> (unsigned 16bit integer=w640:u16)
          n230 = Type Cast(type="", x=w640) -> (*(type *) &x=w642:string)
          n231 = call "7HP_Open serial port.vi"("timeout (ms)"=u32 5000, "VISA resource name"=w635) -> ("Error out"=w636:errorcluster, "VISA resource name out"=w637:refnum<visa-resource-name>)  [unwired: 8 in]
          n232 = Reverse String(1:w642) -> (0:w629:string)
          n233 = call "7HP_Send Cmd + Data.vi"("Error In"=w636, "Data"=w629, "Operation"=w632, "Port"=w637) -> ("Error Out"=w633:errorcluster, "Port out"=w634:refnum<visa-resource-name>)  [unwired: 1 in]
          n234 = call "7HP_Close serial port.vi"("Error in"=w633, "VISA resource name"=w634) -> ("Error out"=w630:errorcluster)  [unwired: 9 in]
        }
        frame #2 {
          n235 = Unbundle By Name(w668) -> ("status"=w669:bool)
          n236 = Not(x=w669) -> (.not. x?=→"sent":bool)
        }
      }
    }
    frame "f" {
      # "Get data rate"
      n237 = flat-sequence {
        tunnel: w679 -> [w683]
        tunnel: [w683] -> w678
        tunnel: w678 -> [w692]
        tunnel: [w695] -> w677
        tunnel: [w697] -> w676
        tunnel: [w703] -> w675
        tunnel: w677 -> [w703]
        tunnel: w676 -> [w701]
        tunnel: [w701] -> w672
        frame #0 {
          n238 = local write "received"(FALSE ("sent")) -> ()
          n239 = local write "Main"(T1."Data rate" ("Main")) -> ()
          n240 = local write "sent"(FALSE ("sent")) -> ()
        }
        frame #1 {
          # "to BE"
          n241 = local read "COM port"() -> (w698:refnum<visa-resource-name>)
          n242 = call "7HP_Open serial port.vi"("timeout (ms)"=u32 5000, "VISA resource name"=w698) -> ("Error out"=w693:errorcluster, "VISA resource name out"=w694:refnum<visa-resource-name>)  [unwired: 8 in]
          n243 = call "7HP_Send Cmd.vi"("Error In"=w693, "Operation"=w692, "Port"=w694) -> ("Error Out"=w690:errorcluster, "Port out"=w689:refnum<visa-resource-name>)  [unwired: 1 in]
          n244 = VISA Read(VISA resource name=w689, byte count=u32 2, error in (no error)=w690) -> (VISA resource name out=w687:refnum<visa-resource-name>, read buffer=w686:string, error out=w688:errorcluster)  [unwired: 1 out]
          n245 = Reverse String(1:w686) -> (0:w696:string)
          n246 = call "7HP_Close serial port.vi"("Error in"=w688, "VISA resource name"=w687) -> ("Error out"=w697:errorcluster)  [unwired: 9 in]
          n247 = Type Cast(type=u16 0 ("byte count"), x=w696) -> (*(type *) &x=w684:u16)
          "Returned data rate (Hz)" <- w684
          n248 = To Double Precision Float(number=w684) -> (double precision float=w695:dbl)
        }
        frame #2 {
          n249 = Unbundle By Name(w701) -> ("status"=w702:bool)
          n250 = Not(x=w702) -> (.not. x?=→"received":bool)
        }
      }
    }
    frame "N" {
      # "Get serial number"
      n251 = flat-sequence {
        tunnel: w707 -> [w712]
        tunnel: [w712] -> w706
        tunnel: w706 -> [w718]
        tunnel: [w717] -> w705
        frame #0 {
          n252 = local write "Main"(T1."Action" ("Main")) -> ()
          "Serial number" <- sgl 0.0 ("Numeric")
        }
        frame #1 {
          # "to BE"
          n253 = local read "COM port"() -> (w719:refnum<visa-resource-name>)
          n254 = call "7HP_Open serial port.vi"("timeout (ms)"=u32 5000, "VISA resource name"=w719) -> ("Error out"=w725:errorcluster, "VISA resource name out"=w726:refnum<visa-resource-name>)  [unwired: 8 in]
          n255 = call "7HP_Send Cmd.vi"("Error In"=w725, "Operation"=w718, "Port"=w726) -> ("Error Out"=w723:errorcluster, "Port out"=w724:refnum<visa-resource-name>)  [unwired: 1 in]
          n256 = VISA Read(VISA resource name=w724, byte count=u32 4, error in (no error)=w723) -> (VISA resource name out=w721:refnum<visa-resource-name>, read buffer=w714:string, error out=w720:errorcluster)  [unwired: 1 out]
          n257 = call "7HP_Close serial port.vi"("Error in"=w720, "VISA resource name"=w721) -> ("Error out"=w717:errorcluster)  [unwired: 9 in]
          n258 = Reverse String(1:w714) -> (0:w715:string)
          n259 = Type Cast(type=sgl 0.0 ("byte count"), x=w715) -> (*(type *) &x=w713:sgl)
          n260 = local write "Serial number"(w713) -> ()
        }
      }
    }
    frame "X" {
      # "Exit"
    }
    frame Default {
    }
  }
  "Data out" <- w2
  "Rendezvous out" <- w1
  n261 = Merge Errors(w12, w11, w10) -> (w9:errorcluster)
  n262 = call <vilib>:"Clear Errors.vi"("error in (no error)"=w9, "specific error code to clear (0: all)"=1073676294) -> ("error out"=w6:errorcluster)  [unwired: 4 in, 1 out]
  n263 = local write "Error"(w6) -> ()
  n264 = Release Queue(queue=w7, error in (no error)=w6) -> (error out=→"Error":errorcluster)  [unwired: 1 in, 2 out]
